vi "AD（V3.2）40M.vi"(8 "N-length":dbl, 9 "M-length":dbl, 10 "hDevice":i32, 11 "pulDDR2Length":u32) -> (0 "幅频谱":dbl[](graph), 1 "时域谱":dbl[](graph), 3 "hDevice out":i32)   [LabVIEW 2016]
uses:
  <vilib>/Analysis/2dsp.llb/Real FFT.vi
  INF/amd64/PCI8502_32.dll
  <vilib>/Analysis/NI_AALPro.lvlib
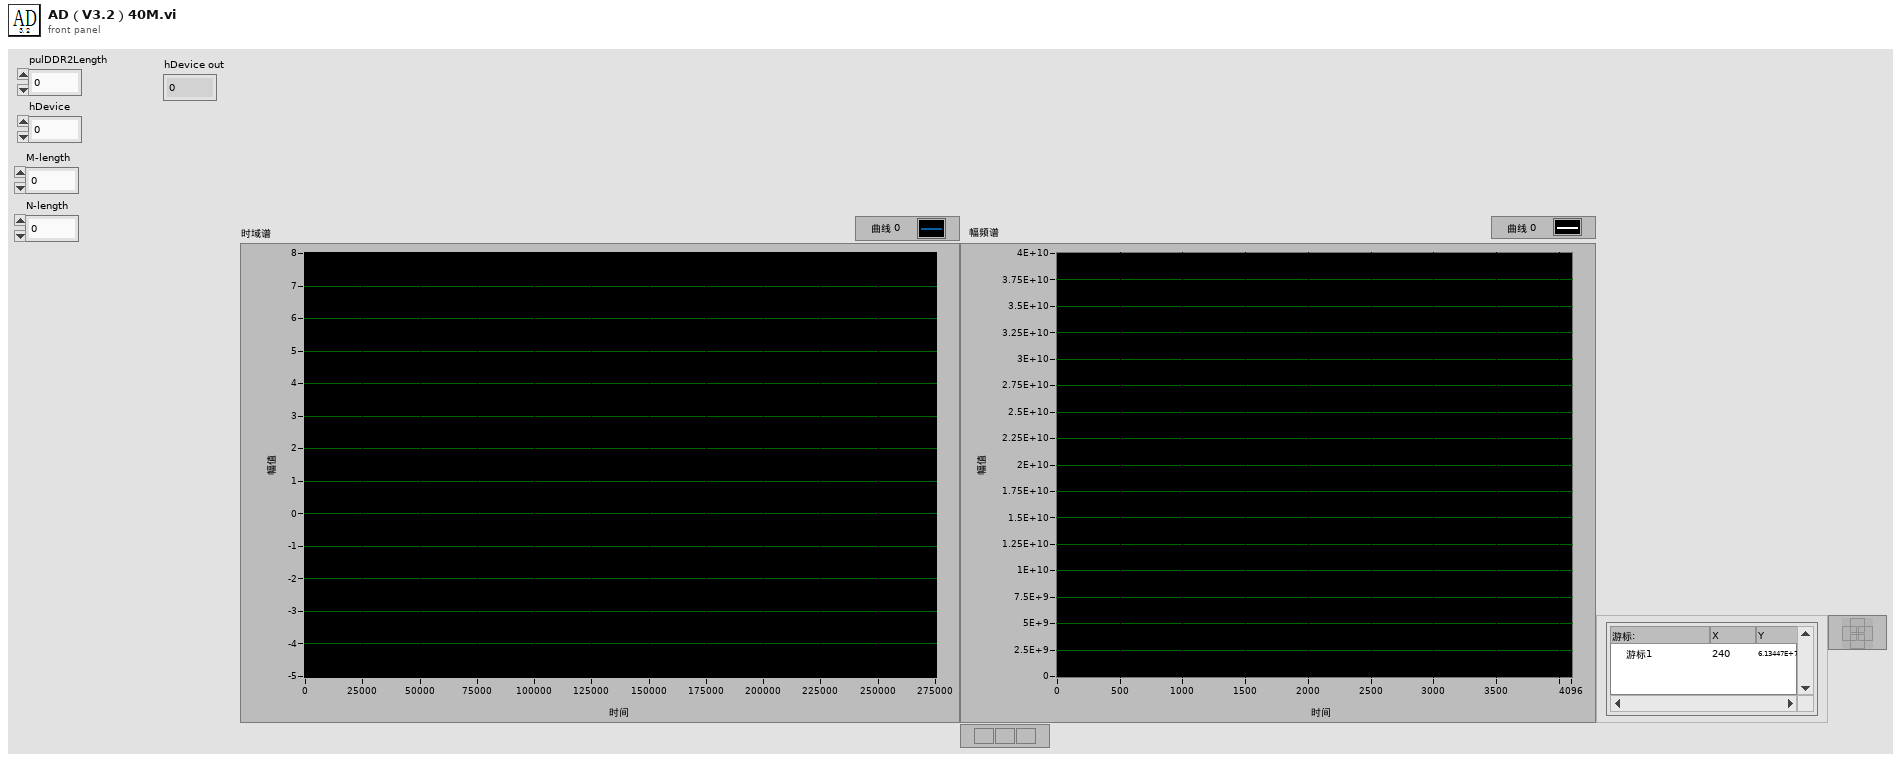
[diagram p1: front panel]
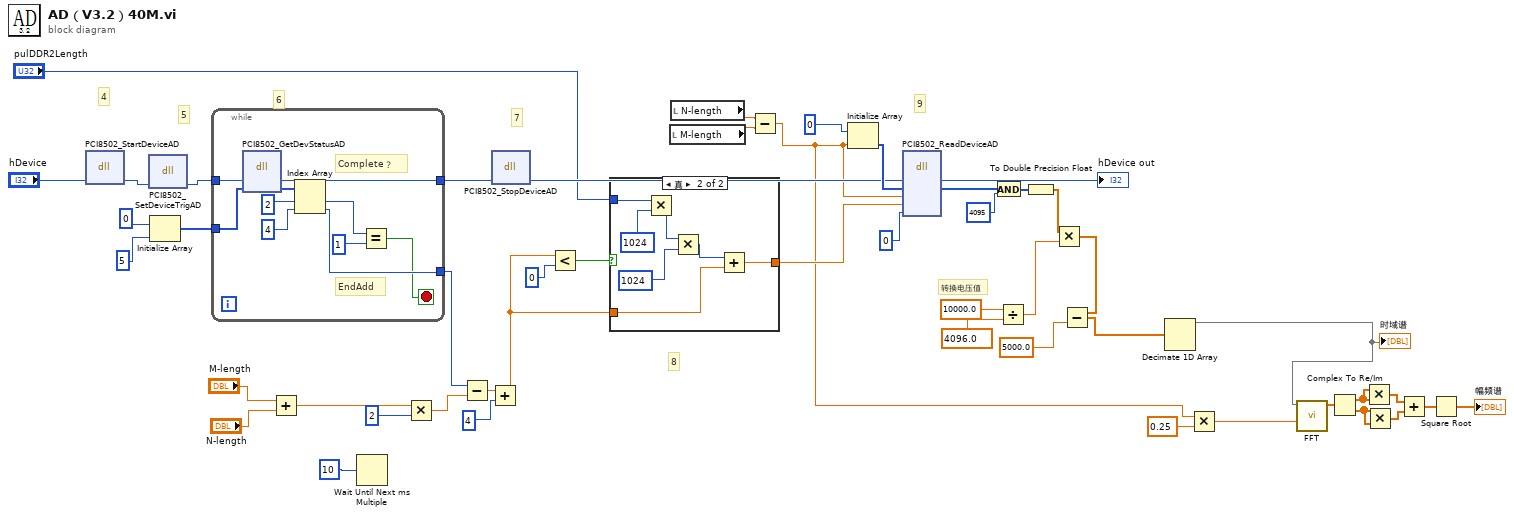
[diagram p0: block diagram]
diagram:
  # "9"
  # "8"
  # "7"
  # "6"
  # "5"
  # "4"
  # "转换电压值"
  n1 = dll-call lib="PTH2]abs CUsersH301Desktopart闭环扫描程序采集卡控制INFamd64\nPCI8502_32" fn="PCI8502_StartDeviceAD" label="StartDeviceAD"("hDevice"="hDevice") -> ("hDevice"=w48:i32)  [unwired: 4 in, 2 out]
  n2 = dll-call lib="PTH2]abs CUsersH301Desktopart闭环扫描程序采集卡控制INFamd64\nPCI8502_32" fn="PCI8502_SetDeviceTrigAD" label="SetDeviceTrigAD"("hDevice"=w48) -> ("hDevice"=w25:i32)  [unwired: 4 in, 2 out]
  n3 = Initialize Array(0, 5) -> (w22:i32[])
  n4 = while {
    tunnel: [w54] -> w21
    tunnel: w25 -> [w53]
    tunnel: w22 -> [w52]
    tunnel: [w51] -> w19
    stop <- w50 stop-if-true
    # "EndAdd"
    # "Complete？"
    n5 = dll-call lib="PTH2aabs CUsersH301Desktopart闭环扫描程序采集卡控制INFamd64PCI8502_32.dll" fn="PCI8502_GetDevStatusAD" label="GetDevStatusAD"("hDevice"=w53, "pADStatus"=w52) -> ("hDevice"=w51:i32, "pADStatus"=w56:i32[])  [unwired: 4 in, 2 out]
    n6 = Index Array(array=w56, index #1=2, index #2=4) -> (element #1=w58:i32, element #2=w54:i32)
    n7 = Equal?(x=w58, y=1) -> (x = y?=w50:bool)
  }
  n8 = Add(x="M-length", y="N-length") -> (x+y=w20:dbl)
  n9 = Wait Until Next ms Multiple(millisecond multiple=u32 10) -> ()  [unwired: 1 out]
  n10 = Multiply(x=w20, y=u32 2) -> (x*y=w33:dbl)
  n11 = Subtract(x=w21, y=w33) -> (x-y=w35:dbl)
  n12 = Add(x=w35, y=u32 4) -> (x+y=w30:dbl)
  n13 = dll-call lib="PTH2]abs CUsersH301Desktopart闭环扫描程序采集卡控制INFamd64\nPCI8502_32" fn="PCI8502_StopDeviceAD" label="StopDeviceAD"("hDevice"=w19) -> ("hDevice"=w36:i32)  [unwired: 4 in, 2 out]
  n14 = Less?(x=w30, y=u32 0) -> (x < y?=w26:bool)
  n15 = case shown="真" w26 {
    tunnel: w30 -> [w60 w63]
    tunnel: [w60 w62] -> w31
    tunnel: "pulDDR2Length" -> [_ w61]
    frame False {
    }
    frame True {
      n16 = Multiply(x=w61, y=u32 1024) -> (x*y=w66:u32)
      n17 = Multiply(x=w66, y=u32 1024) -> (x*y=w64:u32)
      n18 = Add(x=w64, y=w63) -> (x+y=w62:dbl)
    }
  }
  n19 = local read "M-length"() -> (w13:dbl)
  n20 = local read "N-length"() -> (w14:dbl)
  n21 = Subtract(x=w14, y=w13) -> (x-y=w11:dbl)
  n22 = Initialize Array(0, w11) -> (w37:i32[])
  n23 = dll-call lib="PTH2]abs CUsersH301Desktopart闭环扫描程序采集卡控制INFamd64\nPCI8502_32" fn="PCI8502_ReadDeviceAD" label="ReadDeviceAD"("hDevice"=w36, "ADBuffer"=w37, "nReadSizeWords"=w11, "ulStartAddr"=w31, "nRetSizeWords"=0) -> ("hDevice"=→"hDevice out":i32, "ADBuffer"=w28:u16[])  [unwired: 7 in, 2 out]
  n24 = And(x=w28, y=4095) -> (x .and. y?=w39:i32[])
  n25 = Divide(x=10000.0, y=4096.0) -> (x/y=w41:dbl)
  n26 = To Double Precision Float(number=w39) -> (double precision float=w42:dbl[])
  n27 = Multiply(x=w42, y=w41) -> (x*y=w40:dbl[])
  n28 = Subtract(x=w40, y=5000.0) -> (x-y=w2:dbl[])
  n29 = Decimate 1D Array(w2) -> (w1:dbl[])  [unwired: 3 out]
  "时域谱" <- w1
  n30 = Multiply(x=w11, y=0.25) -> (x*y=w10:dbl)
  n31 = call-poly <vilib>:"FFT.vi"("FFT size"=w10, "X"=w1) -> ("FFT {X}"=w9:cdb[])  [unwired: 8 in, 1 out]
  n32 = Complex To Re/Im(x + iy=w9) -> (x=w8:dbl[], y=w7:dbl[])
  n33 = Multiply(x=w8, y=w8) -> (x*y=w6:dbl[])
  n34 = Multiply(x=w7, y=w7) -> (x*y=w5:dbl[])
  n35 = Add(x=w6, y=w5) -> (x+y=w4:dbl[])
  n36 = Square Root(x=w4) -> (sqrt(x)=→"幅频谱":dbl[])
